vi "Validate ipf version and update.vi"(8 "error In":errorcluster, 11 "refnum In":T1) -> (0 "error Out":errorcluster, 3 "refnum Out":T1)   [LabVIEW 2015]
uses:
  <vilib>/Utility/config.llb/Config Data RefNum.ctl
  <vilib>/Utility/config.llb/Read Key (String).vi
  <vilib>/Utility/config.llb/Write Key (String).vi
  <vilib>/Utility/config.llb/Write Key (Path).vi
  <vilib>/Utility/config.llb/NI_LVConfig.lvlib
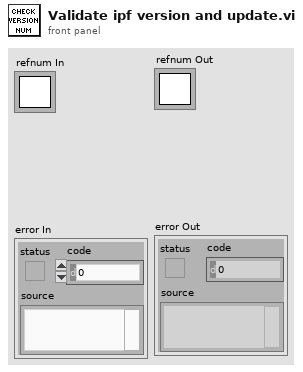
[diagram p1: front panel]
types:
  T1 = typedef "NI_LVConfig.lvlib/Config Data RefNum.ctl" = refnum<k1>
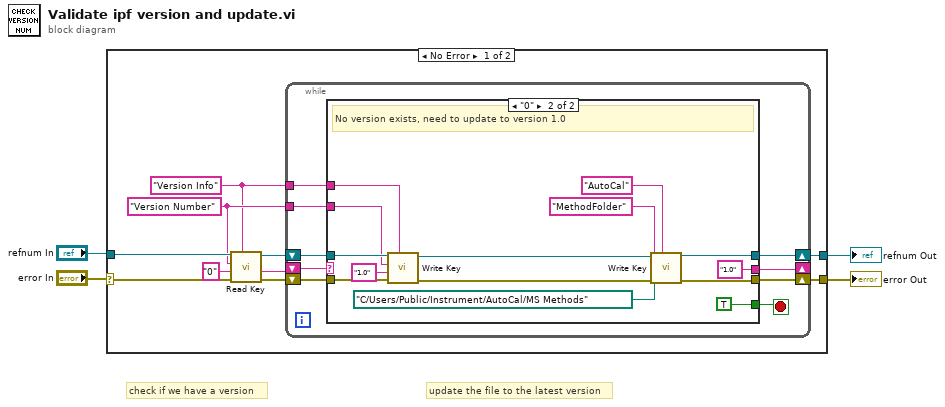
[diagram p0: block diagram]
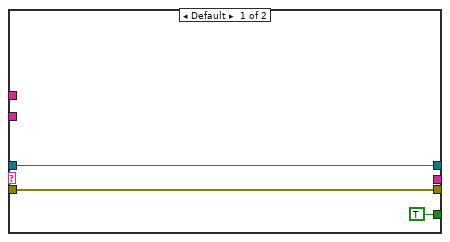
[diagram p2: hidden frame]
diagram:
  # "update the file to the latest version"
  # "check if we have a version"
  n1 = case shown="No Error" "error In" {
    selector: "error In" -> [w14 w42]
    tunnel: [w11 w42] -> w4
    tunnel: "refnum In" -> [w13 w41]
    tunnel: [w9 w41] -> w1
    frame No Error {
      w8 = "Version Number" ("key")
      w7 = "Version Info" ("section")
      n2 = call-poly <vilib>:"Read Key.vi"("section"=w7, "error in (no error)"=w14, "default value"="0", "key"=w8, "refnum"=w13) -> ("error out"=w12:errorcluster, "value"=w5:string, "refnum out"=w10:T1)  [unwired: 3 in, 1 out]
      n3 = while {
        shift-right: [w22] -> w11
        shift-left: w12 -> [w23]
        shift-right: [w20] -> w9
        shift-left: w10 -> [w21]
        shift-right: [w15] -> _
        shift-left: w5 -> [w18]
        tunnel: w8 -> [w16]
        tunnel: w7 -> [w17]
        stop <- w19 stop-if-true
        n4 = case shown="\"0\"" w18 {
          tunnel: w23 -> [w25 w38]
          tunnel: [w25 w32] -> w22
          tunnel: w21 -> [w26 w37]
          tunnel: [w26 w31] -> w20
          tunnel: [TRUE TRUE] -> w19
          tunnel: w17 -> [_ w36]
          tunnel: w16 -> [_ w35]
          tunnel: [_ "1.0" ("value")] -> w15
          frame Default {
          }
          frame "0" {
            # "No version exists, need to update to version 1.0"
            n5 = call-poly <vilib>:"Write Key.vi"("section"=w36, "error in (no error)"=w38, "value"="1.0", "key"=w35, "refnum"=w37) -> ("error out"=w34:errorcluster, "refnum out"=w33:T1)  [unwired: 4 in, 1 out]
            n6 = call-poly <vilib>:"Write Key.vi"("section"="AutoCal", "error in (no error)"=w34, "value"=path "C:/Users/Public/Instrument/AutoCal/MS Methods" ("oldTablePath"), "key"="MethodFolder" ("section"), "refnum"=w33) -> ("error out"=w32:errorcluster, "refnum out"=w31:T1)  [unwired: 4 in, 1 out]
          }
        }
      }
    }
    frame Error {
    }
  }
  "refnum Out" <- w1
  "error Out" <- w4
